vi "randomQuick.vi"() -> ()   [LabVIEW 2018]
uses:
  <userlib>/_OpenG.lib/array/array.llb/Filter 1D Array with Scalar (Boolean)__ogtk.vi
  <userlib>/_OpenG.lib/array/array.llb/Filter 1D Array with Scalar (String)__ogtk.vi
panel:
  out "overCurrent":bool
  out "random":i32
  out "index":i32
  out "Numeric":dbl
  out "?":bool
  out "?":bool
  out "lengthGEA2":i32
  out "lengthRES2":i32
  out "lengthINC2":i32
  out "lengthMPH2":i32
  out "lengthKPH2":i32
  out "GEA2":string[](array[string])
  out "RES2":string[](array[string])
  out "KPH2":string[](array[string])
  out "INC2":string[](array[string])
  out "MPH2":string[](array[string])
  in  "functionQuick":enum16{"PWM", "INC", "RES", "GEA"}(ring)
  out "lengthGEA":i32
  out "lengthRES":i32
  out "lengthINC":i32
  out "lengthKPH":i32
  out "lengthMPH":i32
  out "GEA":string[](array[string])
  out "RES":string[](array[string])
  out "INC":string[](array[string])
  out "KPH":string[](array[string])
  out "MPH":string[](array[string])
  out "graph":dbl(graph)
  out "button":dbl
  out "pass":bool
  out "randomArray":i16[](array[numeric])
  out "max(x,y)":i16
  out "min(x,y)":i16
  out "gauge":dbl(knob) scale=0.0..25.5
  in  "VISA resource name":refnum<visa-resource-name>
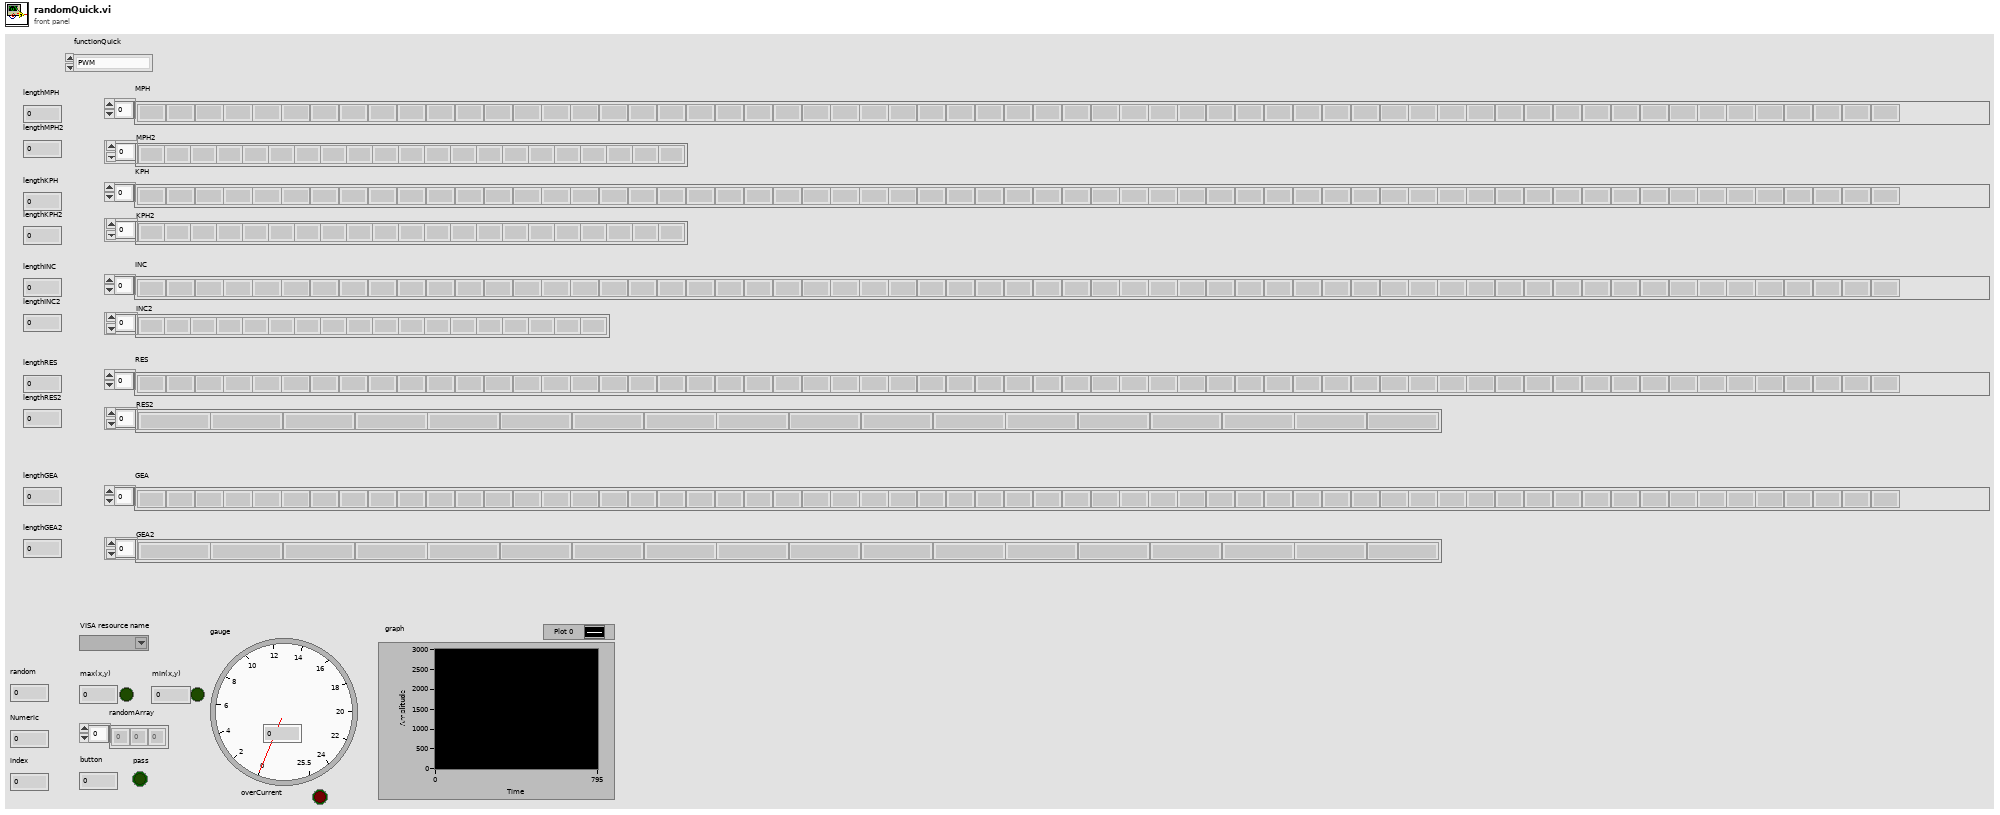
[diagram p1: front panel]
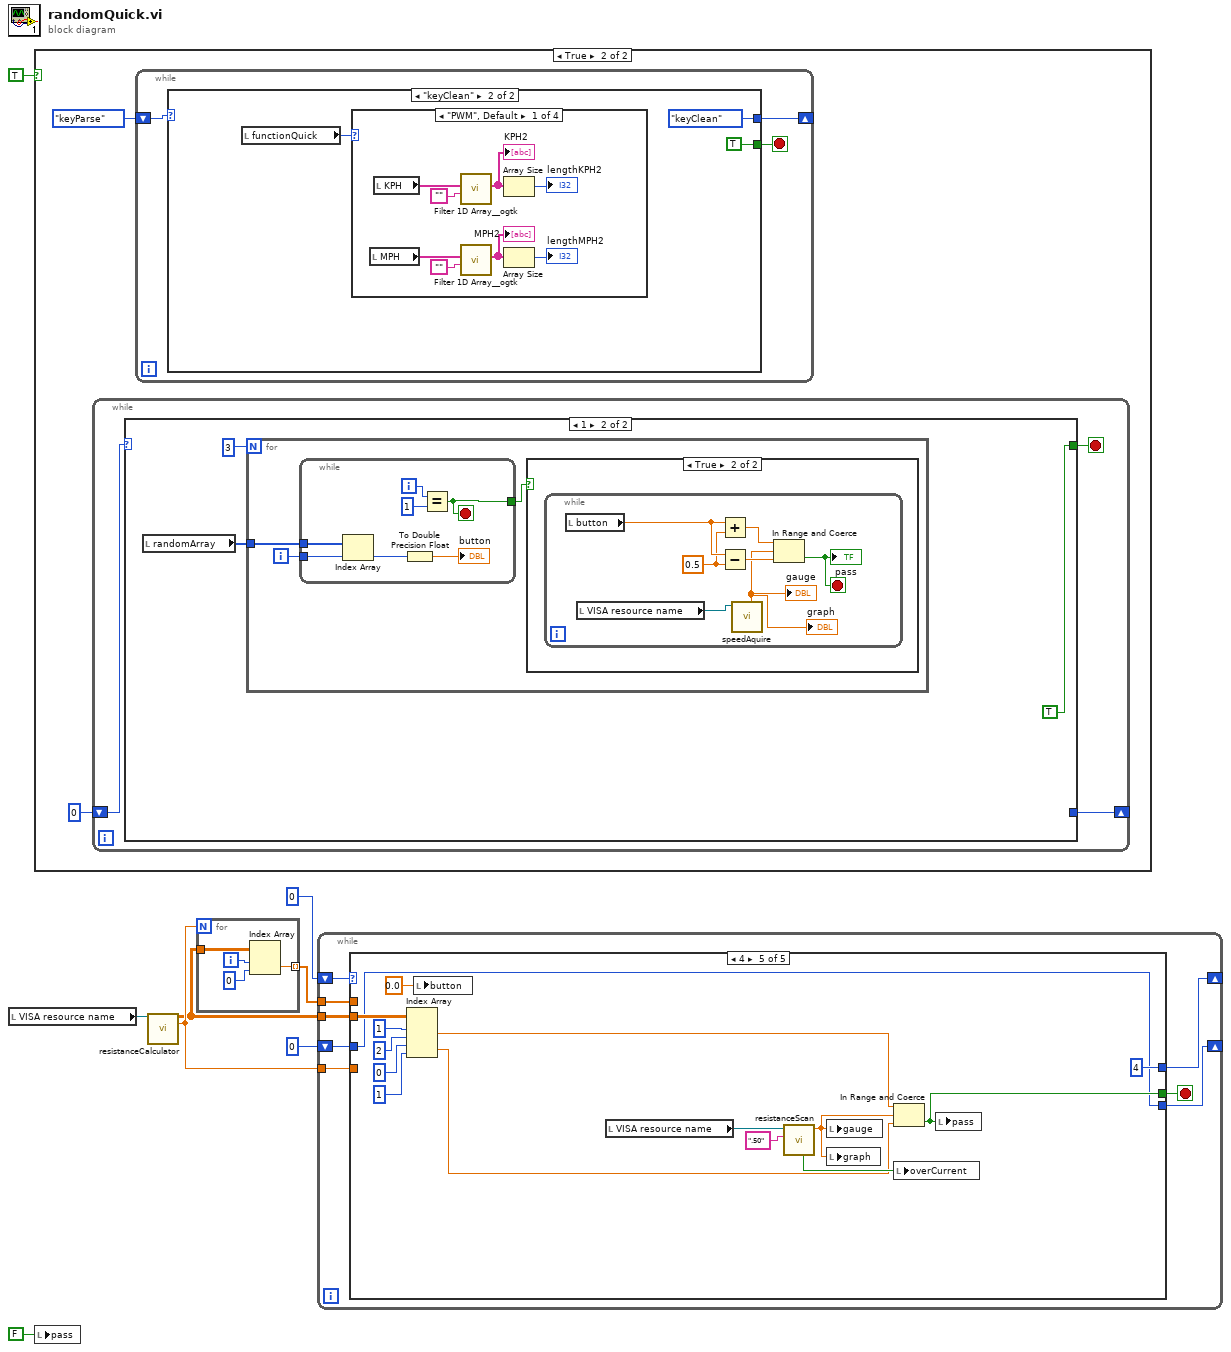
[diagram p0: block diagram]
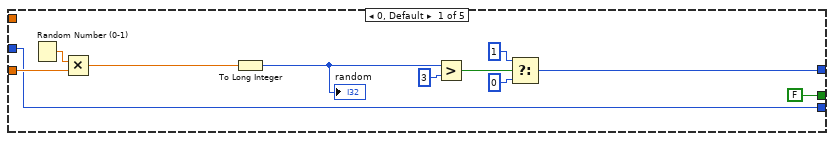
[diagram p2: hidden frame]
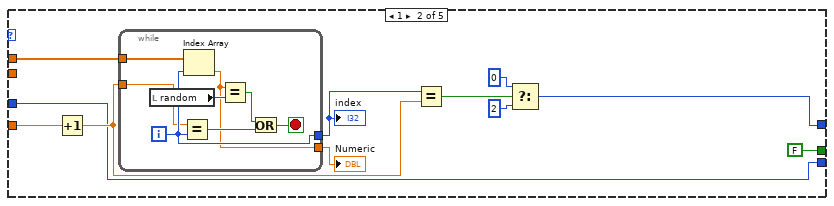
[diagram p3: hidden frame]
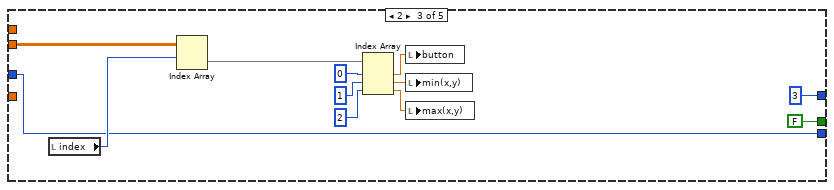
[diagram p4: hidden frame]
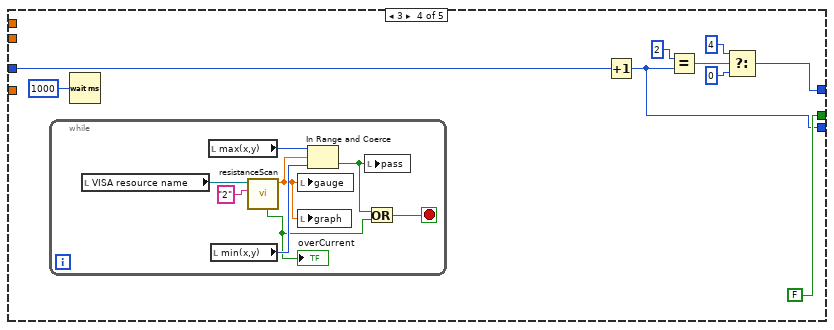
[diagram p5: hidden frame]
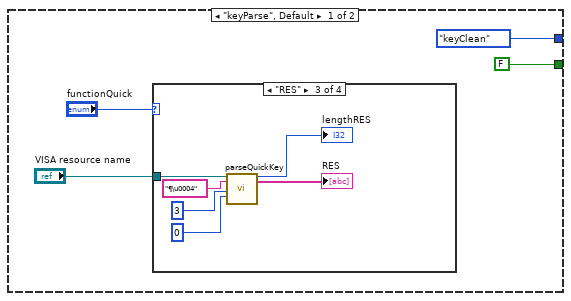
[diagram p7: hidden frame]
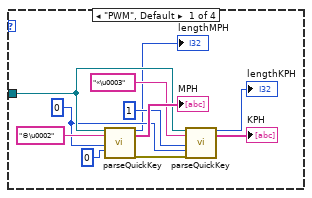
[diagram p8: hidden frame]
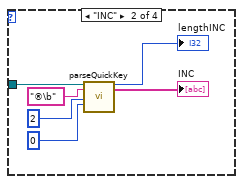
[diagram p9: hidden frame]
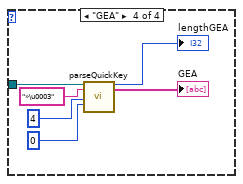
[diagram p10: hidden frame]
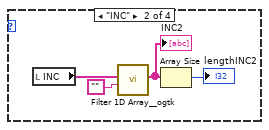
[diagram p11: hidden frame]
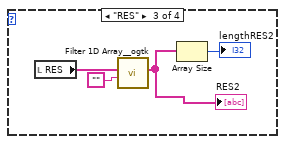
[diagram p12: hidden frame]
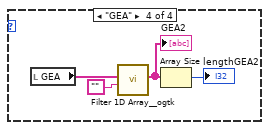
[diagram p13: hidden frame]
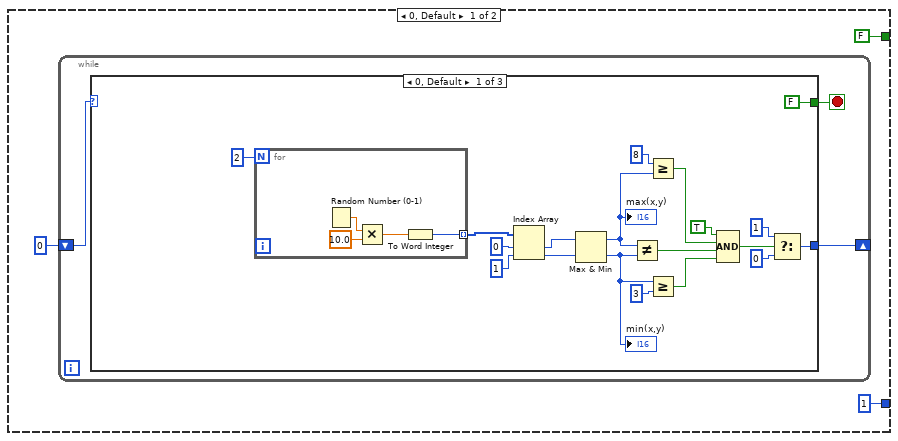
[diagram p14: hidden frame]
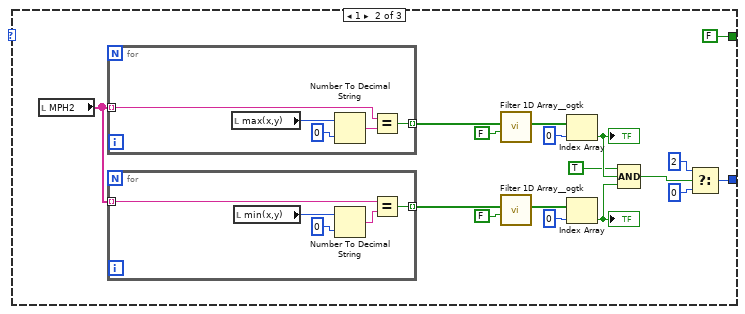
[diagram p15: hidden frame]
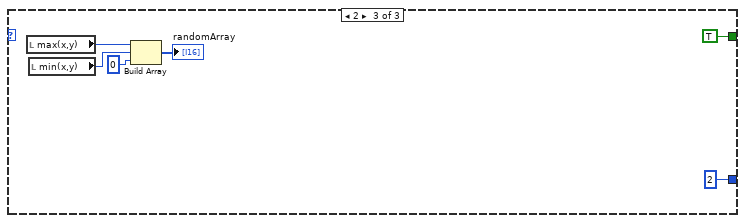
[diagram p16: hidden frame]
diagram:
  n1 = local read "VISA resource name"() -> (w7:refnum<visa-resource-name>)
  n2 = case shown="True" TRUE {
    frame False {
    }
    frame True {
      n3 = while {
        shift-right: [w71] -> _
        shift-left: 0 -> [w72]
        stop <- w70 stop-if-true
        n4 = case shown="1" w72 {
          tunnel: [1 _] -> w71
          tunnel: [FALSE TRUE] -> w70
          frame 0, Default {
            n5 = while {
              shift-right: [w76] -> _
              shift-left: 0 -> [w78]
              stop <- w77 stop-if-true
              n6 = case shown="0, Default" w78 {
                tunnel: [FALSE FALSE TRUE] -> w77
                tunnel: [w79 w104 2 ("f")] -> w76
                frame 0, Default {
                  n7 = for {
                    N: 2 -> [_]
                    tunnel: [w98] -> w97 mode=indexing
                    n8 = Random Number (0-1)() -> (number: 0 to 1=w101:dbl)
                    n9 = Multiply(x=w101, y=10.0) -> (x*y=w99:dbl)
                    n10 = To Word Integer(number=w99) -> (16bit integer=w98:i16)
                  }
                  n11 = Index Array(array=w97, index #1=0 ("index"), index #2=1 ("index")) -> (element #1=w95:i16, element #2=w96:i16)
                  n12 = Max & Min(x=w95, y=w96) -> (max(x,y)=w85:i16, min(x,y)=w91:i16)
                  "max(x,y)" <- w85
                  "min(x,y)" <- w91
                  n13 = Not Equal?(x=w85, y=w91) -> (x != y?=w89:bool)
                  n14 = Greater Or Equal?(x=i16 8 ("y"), y=w85) -> (x >= y?=w87:bool)
                  n15 = Greater Or Equal?(x=w91, y=i16 3) -> (x >= y?=w88:bool)
                  n16 = Compound Arithmetic op=AND(TRUE ("value"), w87, w89, w88) -> (w82:bool)
                  n17 = Select(t=1, s=w82, f=0) -> (s? t:f=w79:i32)
                }
                frame 1 {
                  n18 = local read "MPH2"() -> (w117:string[])
                  n19 = for {
                    tunnel: w117 -> [w128] mode=indexing
                    tunnel: [w124] -> w113 mode=indexing
                    n20 = local read "max(x,y)"() -> (w127:i16)
                    n21 = Number To Decimal String(number=w127, width (-)=i16 0) -> (decimal integer string=w125:string)
                    n22 = Equal?(x=w128, y=w125) -> (x = y?=w124:bool)
                  }
                  n23 = for {
                    tunnel: w117 -> [w123] mode=indexing
                    tunnel: [w119] -> w116 mode=indexing
                    n24 = local read "min(x,y)"() -> (w122:i16)
                    n25 = Number To Decimal String(number=w122, width (-)=i16 0) -> (decimal integer string=w120:string)
                    n26 = Equal?(x=w123, y=w120) -> (x = y?=w119:bool)
                  }
                  n27 = call-poly <userlib>:"Filter 1D Array__ogtk.vi"("items to filter"=FALSE, "array"=w113) -> ("filtered array"=w114:bool[])  [unwired: 4 in, 1 out]
                  n28 = call-poly <userlib>:"Filter 1D Array__ogtk.vi"("items to filter"=FALSE, "array"=w116) -> ("filtered array"=w115:bool[])  [unwired: 4 in, 1 out]
                  n29 = Index Array(array=w114, index=0) -> (element=w108:bool)
                  "?" <- w108
                  n30 = Index Array(array=w115, index=0) -> (element=w107:bool)
                  "?" <- w107
                  n31 = Compound Arithmetic op=AND(TRUE ("value"), w108, w107) -> (w106:bool)
                  n32 = Select(t=2, s=w106, f=0) -> (s? t:f=w104:i32)
                }
                frame 2 {
                  n33 = local read "max(x,y)"() -> (w134:i16)
                  n34 = local read "min(x,y)"() -> (w133:i16)
                  n35 = Build Array(w134, w133, i16 0) -> (→"randomArray":i16[])
                }
              }
            }
          }
          frame 1 {
            n36 = local read "randomArray"() -> (w137:i16[])
            n37 = for {
              N: 3 -> [_]
              tunnel: w137 -> [w140]
              i -> [w139]
              n38 = while {
                tunnel: w140 -> [w154]
                tunnel: w139 -> [w151]
                tunnel: [w148] -> w138
                i -> [w150]
                stop <- w148 stop-if-true
                n39 = Index Array(array=w154, index=w151) -> (element=w153:i16)
                n40 = To Double Precision Float(number=w153) -> (double precision float=→"button":dbl)
                n41 = Equal?(x=w150, y=1) -> (x = y?=w148:bool)
              }
              n42 = case shown="True" w138 {
                frame False {
                }
                frame True {
                  n43 = while {
                    stop <- w143 stop-if-true
                    w146 = 0.5
                    n44 = local read "button"() -> (w147:dbl)
                    n45 = local read "VISA resource name"() -> (w142:refnum<visa-resource-name>)
                    n46 = Add(x=w147, y=w146) -> (x+y=w145:dbl)
                    n47 = Subtract(x=w147, y=w146) -> (x-y=w144:dbl)
                    n48 = call "speedAquire.vi"("VISA resource name"=w142) -> ("SPEED"=w141:dbl)  [unwired: 6 in, 4 out]
                    "gauge" <- w141
                    "graph" <- w141
                    n49 = In Range and Coerce(upper limit=w145, x=w141, lower limit=w144) -> (In Range?=w143:bool)  [unwired: 1 out]
                    "pass" <- w143
                  }
                }
              }
            }
          }
        }
      }
      n50 = while {
        shift-right: [w12] -> _
        shift-left: enum16{"keyParse", "keyClean"}."keyParse" -> [w13]
        stop <- w11 stop-if-true
        n51 = case shown="\"keyClean\"" w13 {
          tunnel: [enum16{"keyParse", "keyClean"}."keyClean" enum16{"keyParse", "keyClean"}."keyClean"] -> w12
          tunnel: [FALSE ("stop") TRUE] -> w11
          frame "keyParse", Default {
            n52 = case shown="\"RES\"" "functionQuick" {
              tunnel: "VISA resource name" -> [w24 w34 w39 w45]
              frame "PWM", Default {
                w22 = 0 ("y")
                n53 = call "parseQuickKey.vi"("VISA resource name"=w24, "write buffer"="©\u0002", "y"=w22, "x"=0) -> ("lengthString"=→"lengthMPH":i32, "KeyCodeName"=→"MPH":string[], "error out"=w23:errorcluster)  [unwired: 11 in, 2 out]
                n54 = call "parseQuickKey.vi"("VISA resource name"=w24, "write buffer"="«\u0003", "y"=1, "x"=w22, "error in (no error)"=w23) -> ("lengthString"=→"lengthKPH":i32, "KeyCodeName"=→"KPH":string[])  [unwired: 10 in, 3 out]
              }
              frame "INC" {
                n55 = call "parseQuickKey.vi"("VISA resource name"=w34, "write buffer"="®\b", "y"=2, "x"=0) -> ("lengthString"=→"lengthINC":i32, "KeyCodeName"=→"INC":string[])  [unwired: 11 in, 3 out]
              }
              frame "RES" {
                n56 = call "parseQuickKey.vi"("VISA resource name"=w39, "write buffer"="¶\u0004", "y"=3, "x"=0) -> ("lengthString"=→"lengthRES":i32, "KeyCodeName"=→"RES":string[])  [unwired: 11 in, 3 out]
              }
              frame "GEA" {
                n57 = call "parseQuickKey.vi"("VISA resource name"=w45, "write buffer"="»\u0003", "y"=4, "x"=0) -> ("lengthString"=→"lengthGEA":i32, "KeyCodeName"=→"GEA":string[])  [unwired: 11 in, 3 out]
              }
            }
          }
          frame "keyClean" {
            n58 = local read "functionQuick"() -> (w49:enum16{"PWM", "INC", "RES", "GEA"})
            n59 = case shown="\"PWM\", Default" w49 {
              frame "PWM", Default {
                n60 = local read "MPH"() -> (w56:string[])
                n61 = local read "KPH"() -> (w55:string[])
                n62 = call-poly <userlib>:"Filter 1D Array__ogtk.vi"("items to filter"="", "array"=w55) -> ("filtered array"=w53:string[])  [unwired: 4 in, 1 out]
                "KPH2" <- w53
                n63 = call-poly <userlib>:"Filter 1D Array__ogtk.vi"("items to filter"="", "array"=w56) -> ("filtered array"=w52:string[])  [unwired: 4 in, 1 out]
                "MPH2" <- w52
                n64 = Array Size(array=w53) -> (size(s)=→"lengthKPH2":i32)
                n65 = Array Size(array=w52) -> (size(s)=→"lengthMPH2":i32)
              }
              frame "INC" {
                n66 = local read "INC"() -> (w61:string[])
                n67 = call-poly <userlib>:"Filter 1D Array__ogtk.vi"("items to filter"="", "array"=w61) -> ("filtered array"=w59:string[])  [unwired: 4 in, 1 out]
                "INC2" <- w59
                n68 = Array Size(array=w59) -> (size(s)=→"lengthINC2":i32)
              }
              frame "RES" {
                n69 = local read "RES"() -> (w65:string[])
                n70 = call-poly <userlib>:"Filter 1D Array__ogtk.vi"("items to filter"="", "array"=w65) -> ("filtered array"=w62:string[])  [unwired: 4 in, 1 out]
                "RES2" <- w62
                n71 = Array Size(array=w62) -> (size(s)=→"lengthRES2":i32)
              }
              frame "GEA" {
                n72 = local read "GEA"() -> (w69:string[])
                n73 = call-poly <userlib>:"Filter 1D Array__ogtk.vi"("items to filter"="", "array"=w69) -> ("filtered array"=w67:string[])  [unwired: 4 in, 1 out]
                "GEA2" <- w67
                n74 = Array Size(array=w67) -> (size(s)=→"lengthGEA2":i32)
              }
            }
          }
        }
      }
    }
  }
  n75 = local write "pass"(FALSE ("pass")) -> ()
  n76 = call "resistanceCalculator.vi"("VISA Refnum in"=w7) -> ("steps/button Array"=w3:dbl[][], "cycle"=w6:dbl)  [unwired: 6 in, 7 out]
  n77 = for {
    N: w6 -> [_]
    tunnel: w3 -> [w158]
    tunnel: [w157] -> w4 mode=indexing
    i -> [w155]
    n78 = Index Array(array=w158, index (row)=w155, index (col)=0) -> (element=w157:dbl)
  }
  n79 = while {
    shift-right: [w165] -> _
    shift-left: 0 -> [w166]
    tunnel: w4 -> [w164]
    tunnel: w6 -> [w163]
    tunnel: w3 -> [w162]
    shift-right: [w160] -> _
    shift-left: 0 -> [w159]
    stop <- w161 stop-if-true
    n80 = case shown="4" w166 {
      tunnel: [w172 w185 3 w211 4 ("f")] -> w165
      tunnel: w164 -> [_ w184 _ _ _]
      tunnel: w163 -> [w171 w180 _ _ _]
      tunnel: w162 -> [_ _ w207 _ w233]
      tunnel: [FALSE FALSE FALSE FALSE w236] -> w161
      tunnel: [w170 w178 w197 w214 w226] -> w160
      tunnel: w159 -> [w170 w178 w197 w216 w226]
      frame 0, Default {
        n81 = Random Number (0-1)() -> (number: 0 to 1=w177:dbl)
        n82 = Multiply(x=w177, y=w171) -> (x*y=w176:dbl)
        n83 = To Long Integer(number=w176) -> (32bit integer=w168:i32)
        "random" <- w168
        n84 = Greater?(x=w168, y=3) -> (0:w169:bool)
        n85 = Select(t=1, s=w169, f=0) -> (s? t:f=w172:i32)
      }
      frame 1 {
        n86 = Increment(x=w180) -> (x+1=w179:dbl)
        n87 = while {
          tunnel: [w193] -> w182
          tunnel: w184 -> [w192]
          tunnel: [w190] -> w183
          tunnel: w179 -> [w189]
          i -> [w193]
          stop <- w194 stop-if-true
          n88 = local read "random"() -> (w191:i32)
          n89 = Equal?(x=w189, y=w193) -> (x = y?=w195:bool)
          n90 = Index Array(array=w192, index=w193) -> (element=w190:dbl)
          n91 = Equal?(x=w190, y=w191) -> (x = y?=w196:bool)
          n92 = Or(x=w196, y=w195) -> (x .or. y?=w194:bool)
        }
        "Numeric" <- w183
        "index" <- w182
        n93 = Equal?(x=w182, y=w179) -> (x = y?=w188:bool)
        n94 = Select(t=0, s=w188, f=2) -> (s? t:f=w185:i32)
      }
      frame 2 {
        n95 = local read "index"() -> (w206:i32)
        n96 = Index Array(array=w207, index (row)=w206) -> (element=w204:dbl[])  [unwired: 1 in]
        n97 = Index Array(array=w204, index #1=0 ("index"), index #2=1 ("index"), index #3=2 ("index")) -> (element #1=w200:dbl, element #2=w198:dbl, element #3=w199:dbl)
        n98 = local write "button"(w200) -> ()
        n99 = local write "min(x,y)"(w198) -> ()
        n100 = local write "max(x,y)"(w199) -> ()
      }
      frame 3 {
        n101 = while {
          stop <- w220 stop-if-true
          n102 = local read "VISA resource name"() -> (w225:refnum<visa-resource-name>)
          n103 = local read "max(x,y)"() -> (w222:i16)
          n104 = local read "min(x,y)"() -> (w223:i16)
          n105 = call "resistanceScan.vi"("Imax"="2", "VISA Refnum in"=w225) -> ("ADC value"=w221:dbl, "overCurrent"=w218:bool)  [unwired: 5 in, 3 out]
          "overCurrent" <- w218
          n106 = local write "gauge"(w221) -> ()
          n107 = local write "graph"(w221) -> ()
          n108 = In Range and Coerce(upper limit=w222, x=w221, lower limit=w223) -> (In Range?=w219:bool)  [unwired: 1 out]
          n109 = local write "pass"(w219) -> ()
          n110 = Or(x=w219, y=w218) -> (x .or. y?=w220:bool)
        }
        n111 = Wait (ms)(milliseconds to wait=u32 1000) -> ()  [unwired: 1 out]
        n112 = Increment(x=w216) -> (x+1=w214:i32)
        n113 = Equal?(x=2, y=w214) -> (x = y?=w209:bool)
        n114 = Select(t=4, s=w209, f=0) -> (s? t:f=w211:i32)
      }
      frame 4 {
        n115 = Index Array(array=w233, index (row) #1=1 ("index (row)"), index (col) #1=2 ("disabled index (col)"), index (row) #2=0 ("disabled index (row)"), index (col) #2=1 ("disabled index (col)")) -> (element #1=w232:dbl, element #2=w231:dbl)
        n116 = local write "button"(0.0 ("button")) -> ()
        n117 = local read "VISA resource name"() -> (w240:refnum<visa-resource-name>)
        n118 = call "resistanceScan.vi"("Imax"=".50", "VISA Refnum in"=w240) -> ("ADC value"=w238:dbl, "overCurrent"=w234:bool)  [unwired: 5 in, 3 out]
        n119 = local write "gauge"(w238) -> ()
        n120 = local write "graph"(w238) -> ()
        n121 = In Range and Coerce(upper limit=w232, x=w238, lower limit=w231) -> (In Range?=w236:bool)  [unwired: 1 out]
        n122 = local write "overCurrent"(w234) -> ()
        n123 = local write "pass"(w236) -> ()
      }
    }
  }
